vi "Execute (Return first result with rows).vi"(8 "error in (no error)":errorcluster, 10 "command":string, 11 "PQ Connection in":refnum<class "PQ Connection.lvclass">) -> (0 "error out":errorcluster, 1 "First Result with Rows returned":refnum<class "PQ Result.lvclass">, 2 "Number of Rows":i32, 3 "PQ Connection out":refnum<class "PQ Connection.lvclass">)   [LabVIEW 2015, in "PQ Connection.lvclass"]
uses:
  PQ Connection.lvclass
  Result/PQ Result.lvclass
  PQ Connection.lvclass/PQ Connection.ctl
  Result/PQ Result.lvclass/PQ Result.ctl
  libpq.dll
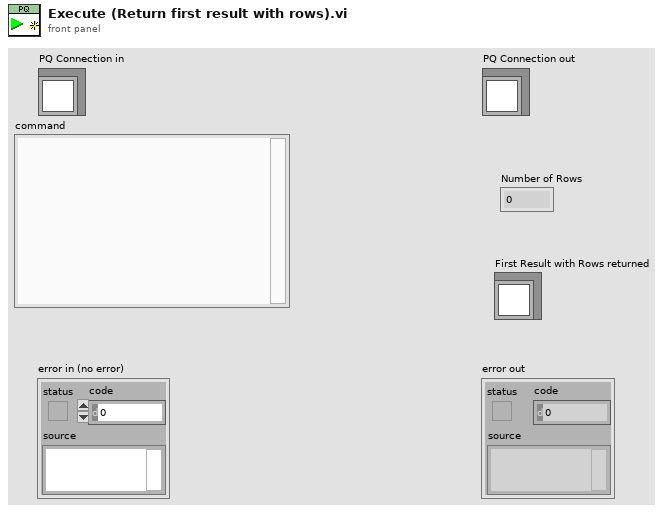
[diagram p1: front panel]
types:
  T1 = typedef "Result Status.ctl" = enum32{"PGRES_EMPTY_QUERY", "PGRES_COMMAND_OK", "PGRES_TUPLES_OK", "PGRES_COPY_OUT", "PGRES_COPY_IN", "PGRES_BAD_RESPONSE", "PGRES_NONFATAL_ERROR", "PGRES_FATAL_ERROR", "PGRES_COPY_BOTH", "PGRES_SINGLE_TUPLE"}
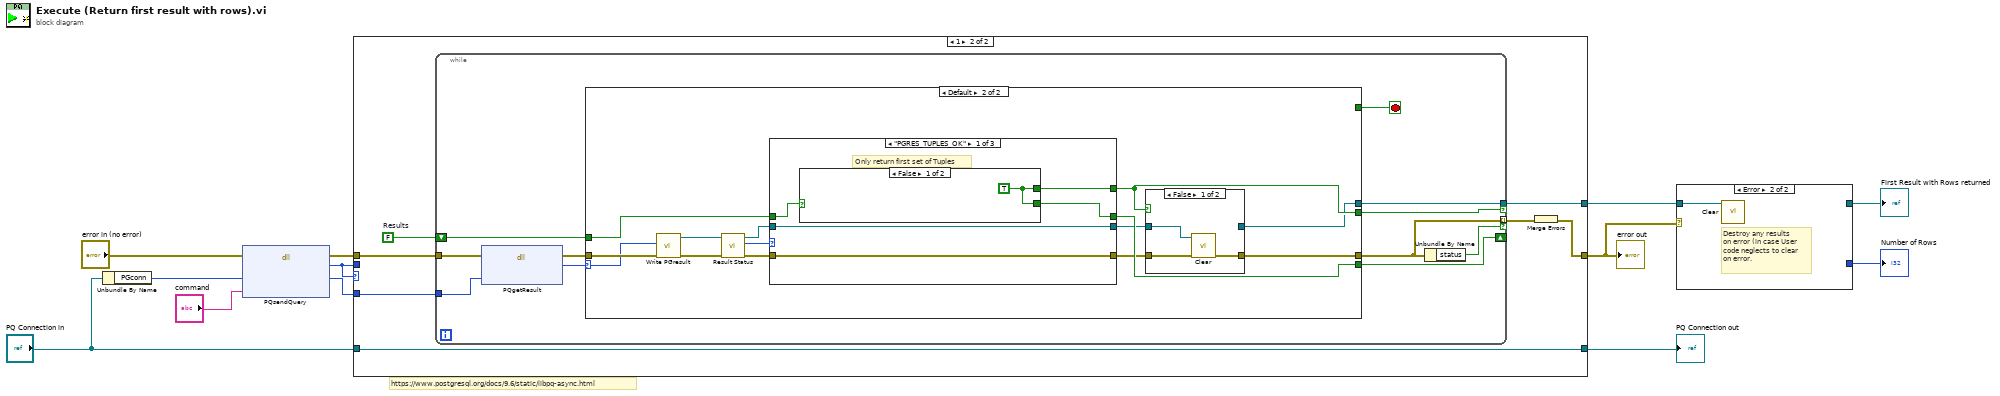
[diagram p0: block diagram]
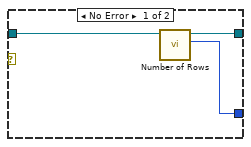
[diagram p2: hidden frame]
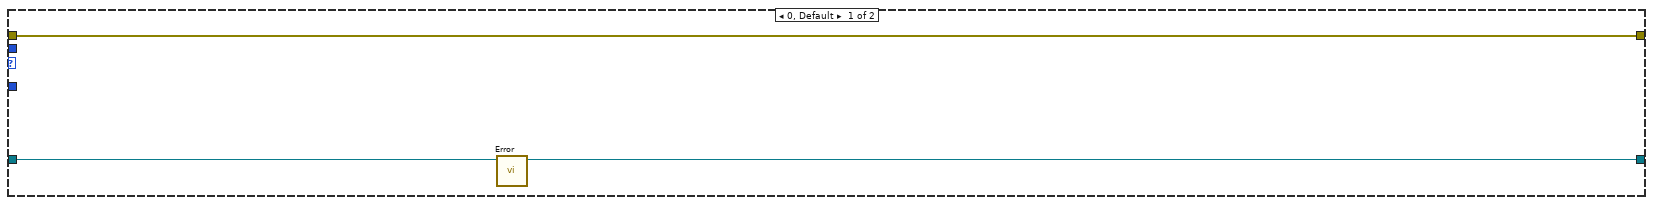
[diagram p3: hidden frame]
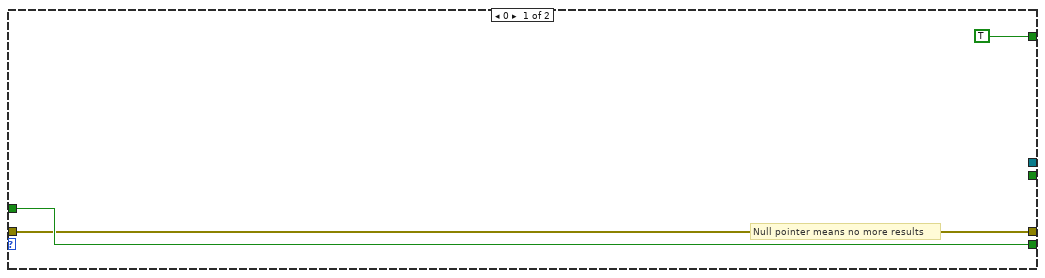
[diagram p4: hidden frame]
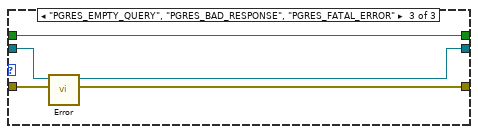
[diagram p7: hidden frame]
diagram:
  # "https://www.postgresql.org/docs/9.6/static/libpq-async.html"
  n1 = Unbundle By Name("PQ Connection in") -> ("PGconn"=w11:u32)
  n2 = dll-call lib="C:/PQ/Connection/libpq.dll" fn="PQsendQuery" ("libpq.*:PQexec")(error in="error in (no error)", "PGconn"=w11, "command"="command") -> (error out=w10:errorcluster, "OK?"=w8:u32, "PGconn"=w5:u32)  [unwired: 3 in, 1 out]
  n3 = case shown="1" w8 {
    tunnel: w10 -> [w13 w22]
    tunnel: w8 -> [_ _]
    tunnel: [_ w21] -> w2
    tunnel: [w13 w16] -> w1
    tunnel: "PQ Connection in" -> [w15 w18]
    tunnel: [w14 w18] -> w6
    tunnel: w5 -> [_ w19]
    frame 0, Default {
      n4 = call "Error.vi"("PQ Connection in"=w15) -> ("PQ Connection out"=w14:refnum<class "PQ Connection.lvclass">)  [unwired: 9 in, 1 out]
    }
    frame 1 {
      w17 = FALSE  # Results
      n5 = while {
        tunnel: [w29] -> w21 if=w30
        tunnel: w19 -> [w33]
        shift-right: [w31] -> _
        shift-left: w17 -> [w32]
        tunnel: w22 -> [w26]
        tunnel: [w24] -> w20 mode=indexing if=w23
        stop <- w27 stop-if-true
        n6 = dll-call lib="C:/PQ/Connection/libpq.dll" fn="PQgetResult" ("libpq.*:PQexec")(error in=w26, "PGconn"=w33) -> (error out=w25:errorcluster, "PQresult"=w28:u32)  [unwired: 3 in, 1 out]
        n7 = case shown="Default" w28 {
          selector: w28 -> [_ w37]
          tunnel: w25 -> [w35 w50]
          tunnel: w32 -> [w36 w49]
          tunnel: [w36 w48] -> w31
          tunnel: [_ w47] -> w30
          tunnel: [_ w45] -> w29
          tunnel: [w35 w43] -> w24
          tunnel: [TRUE _] -> w27
          frame 0 {
            # "Null pointer means no more results"
          }
          frame Default {
            n8 = call "Write PGresult.vi"("error in (no error)"=w50, "PGresult"=w37) -> ("error out"=w41:errorcluster, "PQ Result  out"=w42:refnum<class "PQ Result.lvclass">)  [unwired: 8 in]
            n9 = call "Result Status.vi"("error in (no error)"=w41, "PQ Result in"=w42) -> ("error out"=w38:errorcluster, "Result Status"=w40:T1, "PQ Result out"=w39:refnum<class "PQ Result.lvclass">)  [unwired: 7 in]
            n10 = case shown="\"PGRES_TUPLES_OK\"" w40 {
              tunnel: [w54 w58 w61] -> w46
              tunnel: w39 -> [w54 w58 w65]
              tunnel: w38 -> [w55 w60 w64]
              tunnel: [w55 w60 w62] -> w44
              tunnel: [w53 _ _] -> w47
              tunnel: w49 -> [w52 w59 w63]
              tunnel: [w51 w59 w63] -> w48
              frame "PGRES_TUPLES_OK" {
                # "Only return first set of Tuples"
                n11 = case shown="False" w52 {
                  selector: w52 -> [_ w57]
                  tunnel: [w56 _] -> w53
                  tunnel: [w56 w57] -> w51
                  frame False {
                    w56 = TRUE
                  }
                  frame True {
                  }
                }
              }
              frame Default {
                # "No results, but not error"
              }
              frame "PGRES_EMPTY_QUERY", "PGRES_BAD_RESPONSE", "PGRES_FATAL_ERROR" {
                n12 = call "Error.vi"("error in (no error)"=w64, "PQ Result  In"=w65) -> ("error out"=w62:errorcluster, "PQ Result"=w61:refnum<class "PQ Result.lvclass">)  [unwired: 8 in]
              }
            }
            n13 = case shown="False" w47 {
              tunnel: w46 -> [w68 w70]
              tunnel: [_ w70] -> w45
              tunnel: w44 -> [w67 w69]
              tunnel: [w66 w69] -> w43
              frame False {
                n14 = call "Clear.vi"("error in (no error)"=w67, "PQ Result  in"=w68) -> ("error out"=w66:errorcluster)  [unwired: 9 in]
              }
              frame True {
              }
            }
          }
        }
        n15 = Unbundle By Name(w24) -> ("status"=w23:bool)
      }
      n16 = Merge Errors(w20) -> (w16:errorcluster)
    }
  }
  "error out" <- w1
  "PQ Connection out" <- w6
  n17 = case shown="Error" w1 {
    tunnel: [w73 _] -> w4
    tunnel: [w72 _] -> w3
    tunnel: w2 -> [w71 w74]
    frame No Error {
      n18 = call "Number of Rows.vi"("PQ Result in"=w71) -> ("Number of Rows"=w73:i32, "PQ Result out"=w72:refnum<class "PQ Result.lvclass">)  [unwired: 8 in, 1 out]
    }
    frame Error {
      # "Destroy any results\non error (in case User\ncode neglects to clear\non error."
      n19 = call "Clear.vi"("PQ Result  in"=w74) -> ()  [unwired: 10 in, 1 out]
    }
  }
  "First Result with Rows returned" <- w3
  "Number of Rows" <- w4
